vi "find or create references.vi"(4 "names":string[](array[string]), 6 "paths":path[](array[path]), 7 "vi type":T1, 8 "Data Interface VI":string, 9 "index ctl":string, 10 "data ctl":string, 11 "runtime":refnum<vi>) -> (0 "error out":errorcluster, 3 "vi refs":T2)   [LabVIEW 2013, in "data interface script.lvlib"]
uses:
  data interface script.lvlib
  Controls/initialized references.ctl
  Controls/interface VI type.ctl
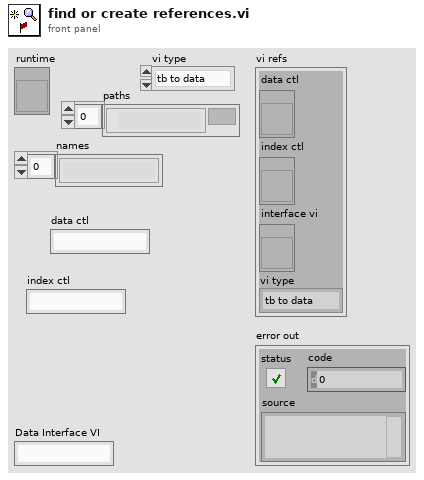
[diagram p1: front panel]
types:
  T1 = typedef "data interface script.lvlib/interface VI type.ctl" = enum16{"tb to data", "data to tb"}
  T2 = typedef "data interface script.lvlib/initialized references.ctl" = cluster{"data ctl":refnum<vi>, "index ctl":refnum<vi>, "interface vi":refnum<vi>, "vi type":T1}
  T3 = enum32{"invalid VI type", "Standard VI", "Control VI", "Global VI", "Polymorphic VI", "Configuration VI", "SubSystem", "Facade VI", "Method VI"}
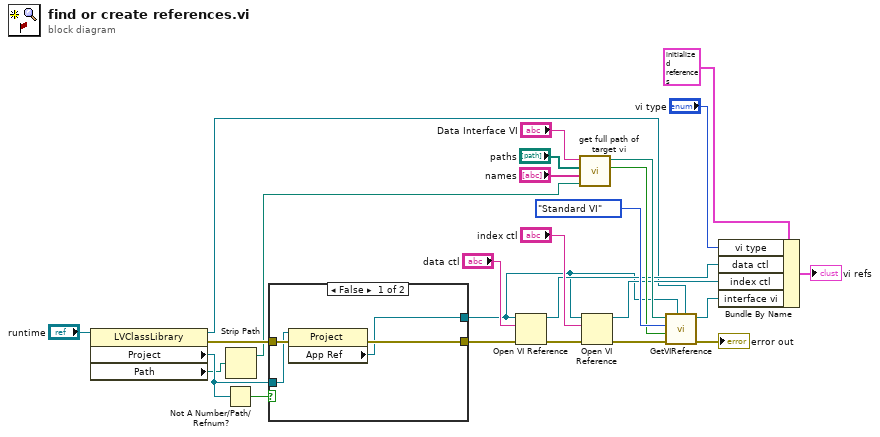
[diagram p0: block diagram]
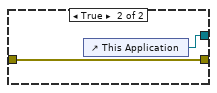
[diagram p2: hidden frame]
diagram:
  n1 = property class="LVClassLibrary"(reference="runtime") -> (reference out=w2:refnum<vi>, error out=w22:errorcluster, "Project"=w21:refnum<vi>, "Path"=w19:path)  [unwired: 1 in]
  n2 = Not A Number/Path/Refnum?(number/path/refnum=w21) -> (NaN/Path/Refnum?=w20:bool)
  n3 = Strip Path(path=w19) -> (stripped path=w17:path)  [unwired: 1 out]
  n4 = case shown="False" w20 {
    tunnel: w22 -> [w30 w32]
    tunnel: [w29 w32] -> w1
    tunnel: w21 -> [w28 _]
    tunnel: [w27 w31] -> w5
    frame False {
      n5 = property class="Project"(reference=w28, error in=w30) -> (error out=w29:errorcluster, "App Ref"=w27:refnum<vi>)  [unwired: 1 out]
    }
    frame True {
      n6 = control-ref of="This Application"() -> (w31:refnum<vi>)
    }
  }
  n7 = Open VI Reference(application reference (local)=w5, vi path="data ctl", error in (no error)=w1) -> (vi reference=w6:refnum<vi>, error out=w10:errorcluster)  [unwired: 3 in]
  n8 = call "get full path of target vi.vi"("class folder path"=w17, "class vi names"="names", "class vi paths"="paths", "vi to qualify"="Data Interface VI") -> ("not in class"=w12:bool, "full path"=w14:path)  [unwired: 6 in]
  n9 = Open VI Reference(application reference (local)=w5, vi path="index ctl", error in (no error)=w10) -> (vi reference=w7:refnum<vi>, error out=w11:errorcluster)  [unwired: 3 in]
  n10 = call "GetVIReference.vi"("LVClassLibrary in"=w2, "application reference"=w5, "error in"=w11, "not in class"=w12, "vi type"=T3."Standard VI", "file path"=w14) -> ("error out"=→"error out":errorcluster, "reference out"=w15:refnum<vi>)  [unwired: 4 in]
  n11 = Bundle By Name(cluster=T2 {"data ctl"=refnum, "index ctl"=refnum, "interface vi"=refnum, "vi type"=enum."tb to data"} ("vi refs"), "vi type"="vi type", "data ctl"=w6, "index ctl"=w7, "interface vi"=w15) -> (→"vi refs":T2)
